vi "wybór wzoru współrzędnych.vi"(4 "Wzory wprowadzanych współrzędnych":u16(ring) items=["D (długość, szerokość)", "D (szerokość, długość)", "DM (długość, szerokość)", "DM (szerokość, długość)", "DMS (długość, szerokość)", "DMS (szerokość, długość)"]) -> (1 "Wzór szukanych współrzędnych punktu":string)   [LabVIEW 2015, in "Biblioteka moduł map v3.lvlib" / "Konwersja wsp.lvlib" / "Wyciągnięcie z tekstu współrzędnej.lvlib"]
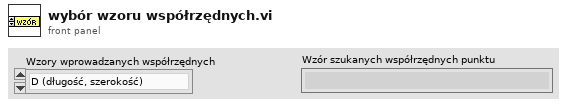
[diagram p1: front panel]
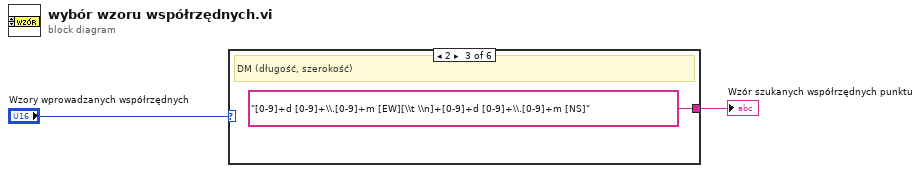
[diagram p0: block diagram]
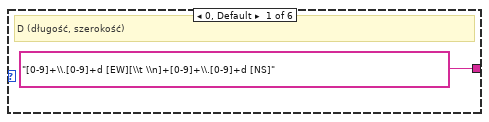
[diagram p2: hidden frame]
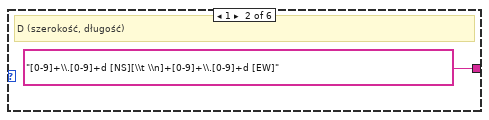
[diagram p3: hidden frame]
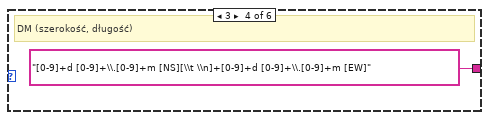
[diagram p4: hidden frame]
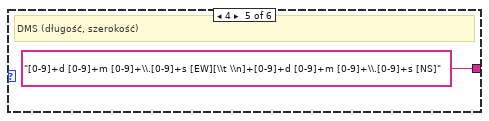
[diagram p5: hidden frame]
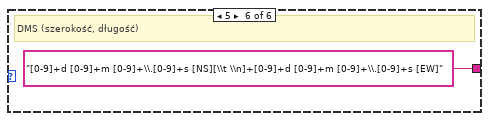
[diagram p6: hidden frame]
diagram:
  n1 = case shown="2" "Wzory wprowadzanych współrzędnych" {
    tunnel: ["[0-9]+\\.[0-9]+d [EW][\\t \\n]+[0-9]+\\.[0-9]+d [NS]" ("regular expression") "[0-9]+\\.[0-9]+d [NS][\\t \\n]+[0-9]+\\.[0-9]+d [EW]" ("regular expression") "[0-9]+d [0-9]+\\.[0-9]+m [EW][\\t \\n]+[0-9]+d [0-9]+\\.[0-9]+m [NS]" ("regular expression") "[0-9]+d [0-9]+\\.[0-9]+m [NS][\\t \\n]+[0-9]+d [0-9]+\\.[0-9]+m [EW]" ("regular expression") "[0-9]+d [0-9]+m [0-9]+\\.[0-9]+s [EW][\\t \\n]+[0-9]+d [0-9]+m [0-9]+\\.[0-9]+s [NS]" ("regular expression") "[0-9]+d [0-9]+m [0-9]+\\.[0-9]+s [NS][\\t \\n]+[0-9]+d [0-9]+m [0-9]+\\.[0-9]+s [EW]" ("regular expression")] -> w1
    frame 0, Default {
      # "D (długość, szerokość)"
    }
    frame 1 {
      # "D (szerokość, długość)"
    }
    frame 2 {
      # "DM (długość, szerokość)"
    }
    frame 3 {
      # "DM (szerokość, długość)"
    }
    frame 4 {
      # "DMS (długość, szerokość)"
    }
    frame 5 {
      # "DMS (szerokość, długość)"
    }
  }
  "Wzór szukanych współrzędnych punktu" <- w1
